vi "_Parse ACLR Result.vi"(8 "error in (no error)":errorcluster, 10 "Input String":string, 11 "VISA resource name":refnum<visa-resource-name>) -> (0 "error out":errorcluster, 1 "Measurement Result":T1 {"NR Pos" format="%^.3e"; "Carrier" format="%^.3e"; "NR Neg" format="%^.3e"}, 2 "Reliability":i32, 3 "VISA resource name out":refnum<visa-resource-name>)   [LabVIEW 2015, in "Rohde&Schwarz CMXP NR FR2 Measurement.lvlib"]
uses:
  <instrlib>/Rohde&Schwarz CMXP NR FR2 Measurement/Rohde&Schwarz CMXP NR FR2 Measurement.lvlib
  <instrlib>/Rohde&Schwarz CMXP NR FR2 Measurement/Private/rsidr_core.llb/rsidr_core.lvlib
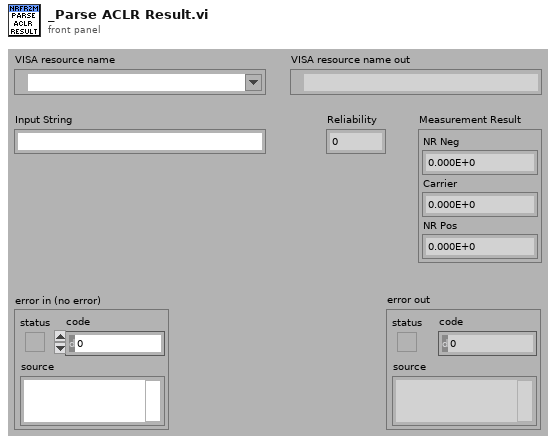
[diagram p1: front panel]
types:
  T1 = cluster{"NR Neg":dbl, "Carrier":dbl, "NR Pos":dbl}
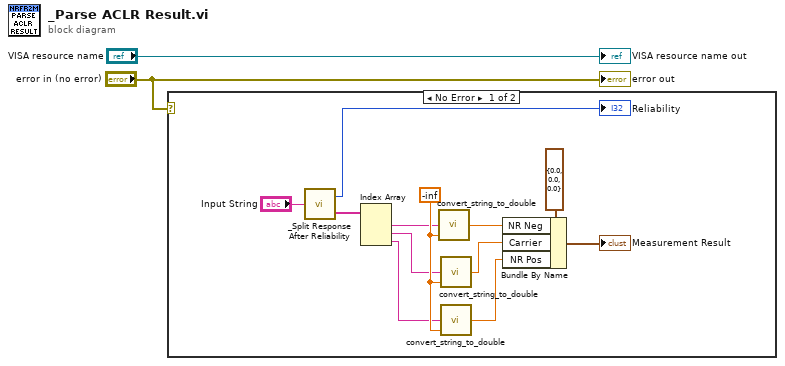
[diagram p0: block diagram]
diagram:
  n1 = case shown="No Error" "error in (no error)" {
    frame No Error {
      w14 = -inf
      n2 = call <instrlib>:"_Split Response After Reliability.vi"("Input String"="Input String") -> ("Response out"=w6:string[], "Reliability out"=→"Reliability":i32)
      n3 = Index Array(array=w6) -> (element #1=w5:string, element #2=w4:string, element #3=w3:string)  [unwired: 3 in]
      n4 = call <instrlib>:"convert_string_to_double.vi"("default (0)"=w14, "String in"=w5) -> ("double value out"=w11:dbl)  [unwired: 3 in]
      n5 = call <instrlib>:"convert_string_to_double.vi"("default (0)"=w14, "String in"=w4) -> ("double value out"=w10:dbl)  [unwired: 3 in]
      n6 = call <instrlib>:"convert_string_to_double.vi"("default (0)"=w14, "String in"=w3) -> ("double value out"=w9:dbl)  [unwired: 3 in]
      n7 = Bundle By Name(cluster=T1 {"NR Neg"=0.0, "Carrier"=0.0, "NR Pos"=0.0} ("Measurement Output"), "NR Neg"=w11, "Carrier"=w10, "NR Pos"=w9) -> (→"Measurement Result":T1)
    }
    frame Error {
    }
  }
  "error out" <- "error in (no error)"
  "VISA resource name out" <- "VISA resource name"
